vi "Execute.vi"(8 "error in (no error)":errorcluster, 9 "System in":refnum<class "System.lvclass">, 10 "Command in":refnum<class "Command.lvclass">, 11 "DM-DFD-Starting-State in":refnum<class "DM-DFD-Starting-State.lvclass">) -> (0 "error out":errorcluster, 2 "Next State":refnum<class "State.lvclass">, 3 "DM-DFD-Starting-State out":refnum<class "DM-DFD-Starting-State.lvclass">)   [LabVIEW 2013, in "DM-DFD-Starting-State.lvclass"]
uses:
  DM-DFD-Starting-State.lvclass
  Commands/Command/Command.lvclass
  Systems/System/System.lvclass
  State/State.lvclass
  Systems/DriveMotors/DriveMotors.lvclass
  DM-DFD-Driving-State/DMD-DFD-Driving-State.lvclass
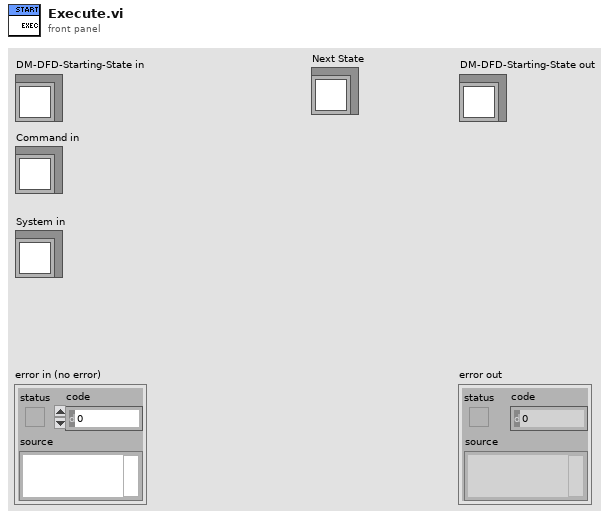
[diagram p1: front panel]
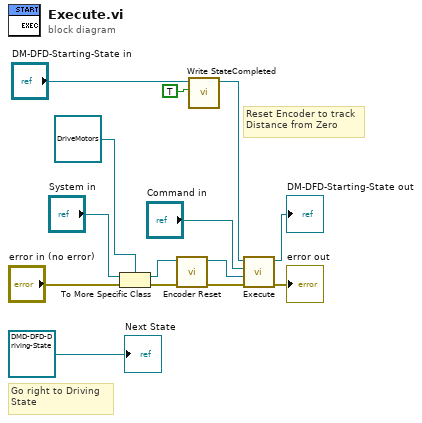
[diagram p0: block diagram]
diagram:
  # "Go right to Driving \nState"
  # "Reset Encoder to track\nDistance from Zero"
  n1 = To More Specific Class(target class=refnum<class "DriveMotors.lvclass"> refnum ("DriveMotors.lvclass"), reference="System in", error in="error in (no error)") -> (specific class reference=w9:refnum<class "DriveMotors.lvclass">, error out=w7:errorcluster)
  n2 = call-dynamic "Encoder Reset.vi"("error in (no error)"=w7, "DriveMotors in"=w9) -> ("error out"=w6:errorcluster, "DriveMotors out"=w4:refnum<class "DriveMotors.lvclass">)  [unwired: 8 in]
  n3 = call-dynamic "Write StateCompleted.vi"("StateCompleted"=TRUE, "State in"="DM-DFD-Starting-State in") -> ("State out"=w2:refnum<class "DM-DFD-Starting-State.lvclass">)  [unwired: 8 in, 1 out]
  n4 = call-parent "Execute.vi"("error in (no error)"=w6, "System in"=w4, "Command in"="Command in", "State in"=w2) -> ("error out"=→"error out":errorcluster, "State out"=→"DM-DFD-Starting-State out":refnum<class "DM-DFD-Starting-State.lvclass">)  [unwired: 5 in, 1 out]
  "Next State" <- refnum<class "DMD-DFD-Driving-State.lvclass"> refnum ("DMD-DFD-Driving-State.lvclass")
